vi "ief_get_extended_status_axis.vi"(0 "Tagprefix in":refnum<k21>, 1 "Axis Number":u16=1 min=1 max=16, 2 "error in (no error)":errorcluster) -> (3 "Tagprefix out":refnum<k21>, 4 "Extended Axis State Cluster":T1, 5 "Extended Axis State":u32, 6 "error out (no error)":errorcluster)   [LabVIEW 2015, in "IEF Werner.lvlib"]
doc: "The VI returns the present extended axis state of the chosen axis as a real number as well as a state cluster.\n\nAxis Number Range:\n01, 10 hex\n1, 16 dec"
uses:
  IEF Werner.lvlib
  ief_xxu/ief_extended_status_axis_cluster.ctl
panel:
  in  "Extended Axis State Cluster in":T1
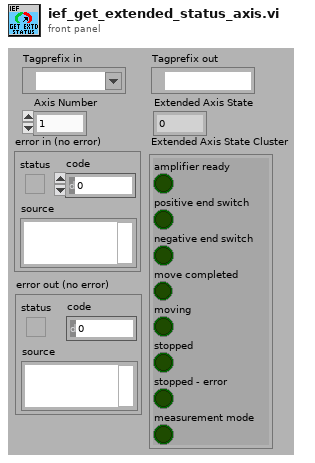
[diagram p1: front panel]
types:
  T1 = typedef "IEF Werner.lvlib/ief_extended_status_axis_cluster.ctl" = cluster{"amplifier ready":bool, "positive end switch":bool, "negative end switch":bool, "move completed":bool, "moving":bool, "stopped":bool, "stopped - error ":bool, "measurement mode":bool}
  T2 = typedef "Semaphore RefNum" = refnum<k1>
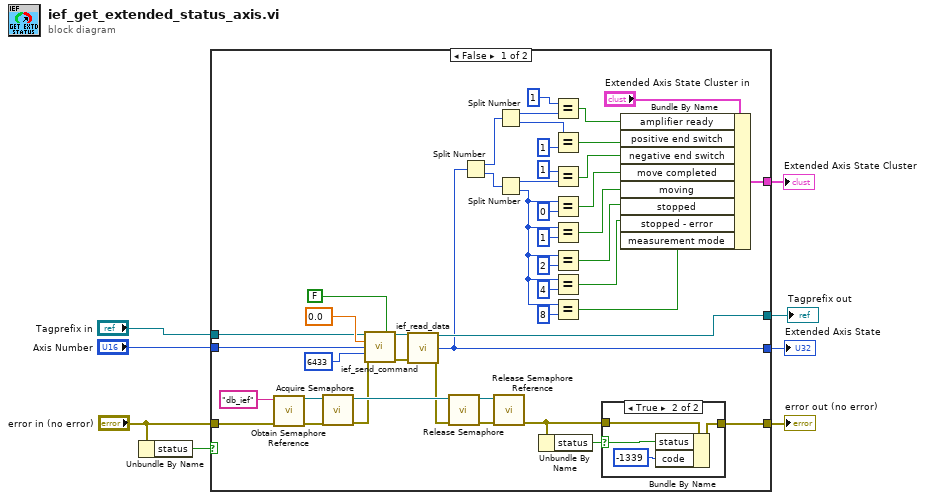
[diagram p0: block diagram]
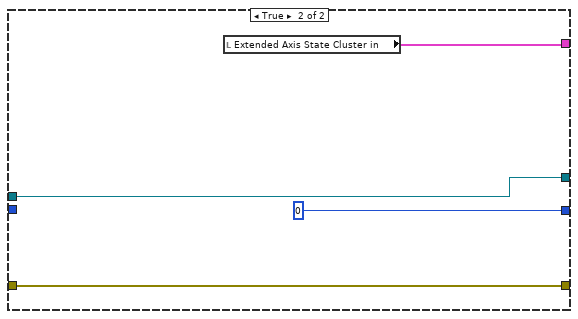
[diagram p3: hidden frame]
diagram:
  n1 = Unbundle By Name("error in (no error)") -> ("status"=w5:bool)
  n2 = case shown="False" w5 {
    tunnel: "Axis Number" -> [w51 _]
    tunnel: "error in (no error)" -> [w42 w62]
    tunnel: [w49 w62] -> w7
    tunnel: [w9 u32 0 ("value uint 32")] -> w4
    tunnel: [w13 w60] -> w3
    tunnel: "Tagprefix in" -> [w12 w61]
    tunnel: [w10 w61] -> w1
    frame False {
      n3 = call <vilib>:"Obtain Semaphore Reference.vi"("error in (no error)"=w42, "name (unnamed)"="db_ief") -> ("error out"=w46:errorcluster, "semaphore"=w47:T2)  [unwired: 3 in, 1 out]
      n4 = call <vilib>:"Acquire Semaphore.vi"("error in (no error)"=w46, "semaphore"=w47) -> ("error out"=w41:errorcluster, "semaphore out"=w45:T2)  [unwired: 3 in, 1 out]
      n5 = call "ief_send_command.vi"("Tagprefix in"=w12, "Command datum of type real"=FALSE, "Command datum"=sgl 0.0, "Command parameter"=w51, "Command code"=u16 6433, "error in (no error)"=w41) -> ("Tagprefix out"=w11:refnum<k21>, "error out (no error)"=w50:errorcluster)  [unwired: 4 in, 4 out]
      n6 = call "ief_read_data.vi"("Tagprefix in"=w11, "error in (no error)"=w50) -> ("Tagprefix out"=w10:refnum<k21>, "value uint 32"=w9:u32, "error out (no error)"=w40:errorcluster)  [unwired: 7 in, 4 out]
      n7 = call <vilib>:"Release Semaphore.vi"("error in (no error)"=w40, "semaphore"=w45) -> ("error out"=w44:errorcluster, "semaphore out"=w43:T2)  [unwired: 4 in]
      n8 = Split Number(x=w9) -> (hi(x)=w35:u16, lo(x)=w36:u16)
      n9 = call <vilib>:"Release Semaphore Reference.vi"("error in (no error)"=w44, "semaphore"=w43) -> ("error out"=w39:errorcluster)  [unwired: 8 in, 1 out]
      n10 = Split Number(x=w35) -> (hi(x)=w33:u8, lo(x)=w28:u8)
      n11 = Split Number(x=w36) -> (hi(x)=w26:u8, lo(x)=w25:u8)
      n12 = Unbundle By Name(w39) -> ("status"=w38:bool)
      n13 = Equal?(x=u8 1, y=w33) -> (x = y?=w31:bool)
      n14 = Equal?(x=w28, y=u8 1) -> (x = y?=w29:bool)
      n15 = Equal?(x=u8 1 ("y"), y=w26) -> (x = y?=w19:bool)
      n16 = Equal?(x=w25, y=u8 0) -> (x = y?=w18:bool)
      n17 = Equal?(x=w25, y=u8 1) -> (x = y?=w17:bool)
      n18 = Equal?(x=w25, y=u8 2) -> (x = y?=w16:bool)
      n19 = Equal?(x=w25, y=u8 4) -> (x = y?=w15:bool)
      n20 = Equal?(x=w25, y=u8 8) -> (x = y?=w14:bool)
      n21 = case shown="True" w38 {
        selector: w38 -> [_ w55]
        tunnel: [w54 w57] -> w49
        tunnel: w39 -> [w54 w58]
        frame False {
        }
        frame True {
          n22 = Bundle By Name(cluster=w58, "status"=w55, "code"=-1339) -> (w57:errorcluster)
        }
      }
      n23 = Bundle By Name(cluster="Extended Axis State Cluster in", "amplifier ready"=w31, "positive end switch"=w29, "negative end switch"=w19, "move completed"=w18, "moving"=w17, "stopped"=w16, "stopped - error"=w15, "measurement mode"=w14) -> (w13:T1)
    }
    frame True {
      n24 = local read "Extended Axis State Cluster in"() -> (w60:T1)
    }
  }
  "error out (no error)" <- w7
  "Extended Axis State" <- w4
  "Extended Axis State Cluster" <- w3
  "Tagprefix out" <- w1
